vi "viayka.vi"(8 "Num":i16, 11 "Array":T2(array[cluster])) -> (0 "Num Out":i32)   [LabVIEW 2020]
uses:
  Action control.ctl
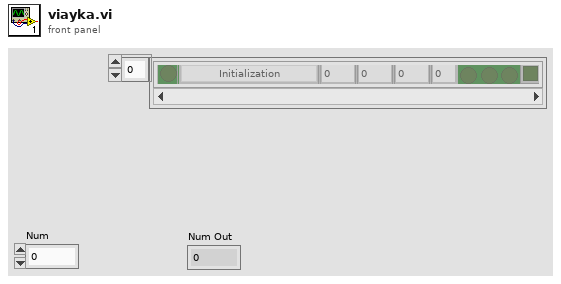
[diagram p1: front panel]
types:
  T1 = typedef "Action control.ctl" = enum16{"Initialization", "Start", "Smooth pause", "autonomus", "Pause", "Camera", "Rotation", "Rotation Correct", "Move", "Move GPS", "Lift", "OMS", "Gamepad", "Go to", "Empty script", "Run scripts", "End"}
  T2 = cluster{"Activ":bool, "X":dbl, "Y":dbl, "Z":dbl, "Div":i8, "Set 1":bool, "Set 2":bool, "Set 3":bool, "Skip":bool, "action":T1}[]
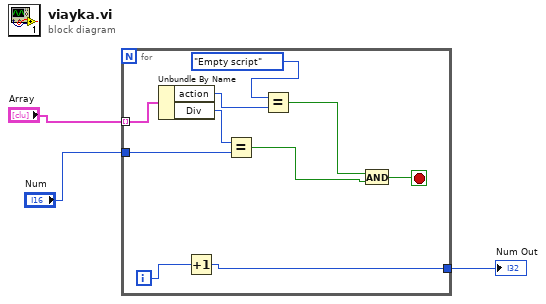
[diagram p0: block diagram]
diagram:
  n1 = for {
    tunnel: "Array" -> [w13] mode=indexing
    tunnel: "Num" -> [w6]
    tunnel: [w4] -> w1
    i -> [w5]
    stop <- w12 stop-if-true
    n2 = Unbundle By Name(w13) -> ("action"=w10:T1, "Div"=w9:i8)
    n3 = Increment(x=w5) -> (x+1=w4:i32)
    n4 = Equal?(x=w9, y=w6) -> (x = y?=w8:bool)
    n5 = Equal?(x=Action_control."Empty script" ("action"), y=w10) -> (x = y?=w7:bool)
    n6 = And(x=w7, y=w8) -> (x .and. y?=w12:bool)
  }
  "Num Out" <- w1
